vi "ModuleTest_3614.vi"() -> ()   [LabVIEW 2012]
panel:
  out "Output":T1
  out "output":string
  in  "input":string
  in  "布尔":bool
  out "error out":errorcluster caption="错误输出"
  in  "停止":bool
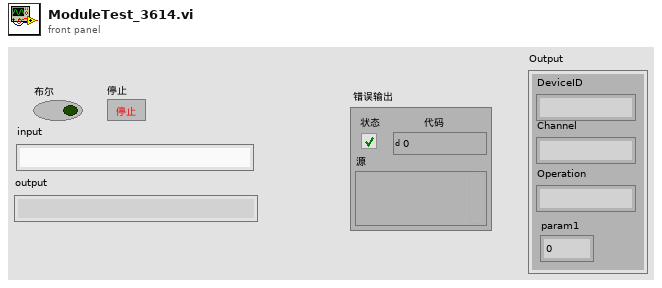
[diagram p1: front panel]
types:
  T1 = cluster{"DeviceID":string, "Channel":string, "param1":dbl, "Operation":string}
  T2 = cluster{"ref_out":cluster{bool, "Conn. Axes out":string[]}, "ref_out":cluster{"ref_type":cluster{"MG17Motor":refnum<k7>, "MG17Motor 2":refnum<k7>, "MG17Motor 3":refnum<k7>, "MG17Motor 4":refnum<k7>, "MG17Motor 5":refnum<k7>, "MG17Motor 6":refnum<k7>}, bool[]}, "ref_out":cluster{"AG-UC2-UC8 Reference":refnum<k24>, "Instrument Key OUT":string, "Error":i32, "REDY":bool}, "ref_out":cluster{"CmdLib Out":refnum<k24>, "DeviceKey Out":string, "Device Address":i32, "REDY":bool}}
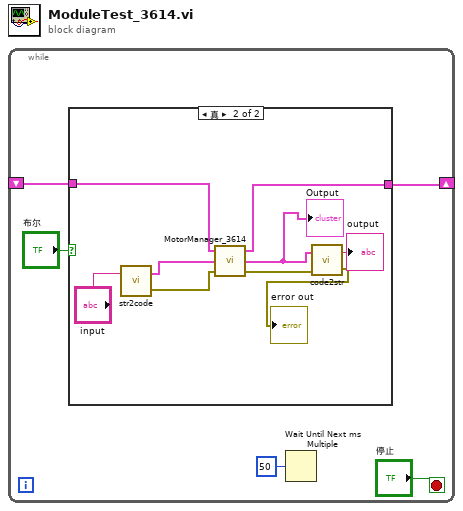
[diagram p0: block diagram]
diagram:
  n1 = while {
    shift-right: [w3] -> _
    shift-left: _ -> [w2]
    stop <- "停止" stop-if-true
    n2 = case shown="真" "布尔" {
      tunnel: [w6 w9] -> w3
      tunnel: w2 -> [w6 w8]
      frame False {
      }
      frame True {
        n3 = call "str2code.vi"("input"="input") -> ("error out"=w14:errorcluster, "Output"=w15:T1)  [unwired: 1 in]
        n4 = call "MotorManager_3614.vi"("error in (no error)"=w14, "Input"=w15, "ref_in"=w8) -> ("error out"=w12:errorcluster, "Output"=w7:T1, "ref_out"=w9:T2)
        "Output" <- w7
        n5 = call "code2str.vi"("错误输入"=w12, "input"=w7) -> ("error out"=→"error out":errorcluster, "output"=→"output":string)
      }
    }
    n6 = Wait Until Next ms Multiple(millisecond multiple=u32 50 ("毫秒倍数")) -> ()  [unwired: 1 out]
  }
